vi "icl_update_test.vi"   [LabVIEW 2018]
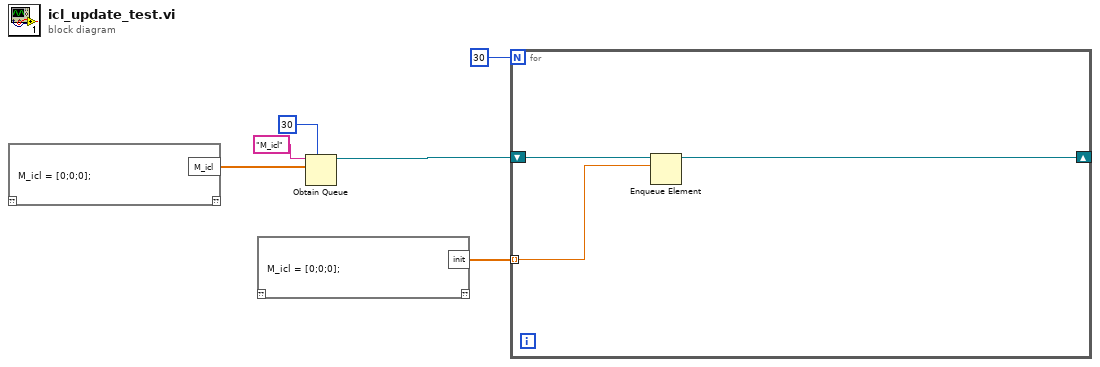
[diagram p0: block diagram]
diagram:
  n1 = mathscript code="M_icl = [0;0;0];"() -> ("M_icl"=w5:dbl[])  [unwired: 1 in, 1 out]
  n2 = mathscript code="M_icl = [0;0;0];"() -> ("init"=w1:dbl[])  [unwired: 1 in, 1 out]
  n3 = Obtain Queue(max queue size (-1, unlimited)=30, name (unnamed)="M_icl", element data type=w5) -> (queue out=w2:refnum<queue>)  [unwired: 2 in, 2 out]
  n4 = for {
    N: 30 -> [_]
    shift-right: [w8] -> _
    shift-left: w2 -> [w9]
    tunnel: w1 -> [w7] mode=indexing
    n5 = Enqueue Element(queue=w9, element=w7) -> (queue out=w8:refnum<queue>)  [unwired: 2 in, 2 out]
  }
